vi "niFPGA Resampler Output Buffer.vi"(8 "wrEn":bool, 9 "wrVal":fxp<+/-,18,1>, 10 "ready for output":bool, 11 "reset":bool) -> (0 "wrTimedOut?":bool, 1 "rdTimedOut?":bool, 2 "outputValid":bool, 3 "outputData":fxp<+/-,18,1> format="%.18g")   [LabVIEW 2017]
uses:
  <vilib>/rvi/Emulation/niFpgaSctlEmulationGetInTimedLoop.vi
  <vilib>/Utility/error.llb/Clear Errors.vi
  <vilib>/rvi/DataTransferAndStorage/Container/Common/niFpgaContainerGetUniqueNameForEmu.vi
  <vilib>/rvi/DataTransferAndStorage/Container/Common/niFpgaContainerSetEmuInfo.vi
  <vilib>/rvi/eio/common/nirviEmuReportErrorAndStop.vi
  <vilib>/rvi/DataTransferAndStorage/Container/Common/niFpgaContainerExecOnDevCompGetState.vi
  <vilib>/rvi/Emulation/niFpgaEmulationIsFPGAContextNoSignature.vi
  <vilib>/rvi/errors/niFpgaSetErrorForExecOnDevCompSimple.vi
  <vilib>/rvi/FIFO/Fifo_Resource/nirvififoEmulationSetSize.vi
  <vilib>/rvi/FIFO/Fifo_Resource/nirviFifoEmulationQueueMgr.vi
  <instcachedir>/0/nirviFifoEmulationQueueMgr_E5CAEC123FF24DC58D834DCA3CDAA9B5.lvgen/nirviFifoEmulationQueueMgr_E5CAEC123FF24DC58D834DCA3CDAA9B5_002.vi
  <vilib>/rvi/FIFO/Fifo_Resource/nirvififoEmulationDetermineInputValidOut.vi
  <vilib>/rvi/FIFO/Fifo_Resource/nirvififoEmulationCreateLock.vi
  <vilib>/rvi/Emulation/niFpgaProcessEmulError.vi
  <vilib>/rvi/FIFO/Fifo_Resource/nirvififoEmulationObtainLock.vi
  <vilib>/rvi/FIFO/Fifo_Resource/nirvififoEmulationReleaseLock.vi
  <vilib>/rvi/occurrence/nirviWaitOnOccurrenceBase.vi
  <vilib>/rvi/errors/nirviReportUnexpectedCaseInternalError.vi
  <vilib>/rvi/errors/nirviReportUnexpectedCaseInternalError (U32).vi
  <vilib>/rvi/interface/RandomDataEmulation/niFpgaRandomDataHandleErrors.vi
  <vilib>/rvi/LocalResourceManager/LocalResourceManager.xnode
  <vilib>/rvi/DataTransferAndStorage/Container/XNode/niFpgaContainer.xnode
  <vilib>/rvi/FIFO/Fifo_Resource/niFpgaFifoEmulationRefIn.vi
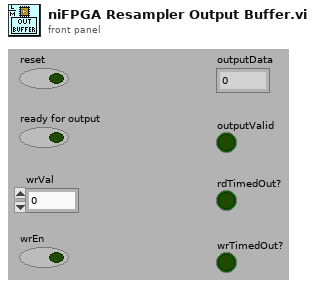
[diagram p1: front panel]
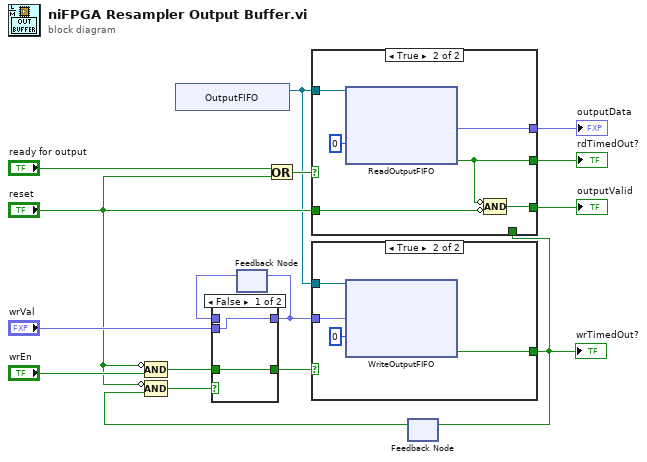
[diagram p0: block diagram]
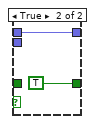
[diagram p2: hidden frame]
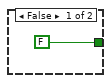
[diagram p3: hidden frame]
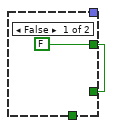
[diagram p4: hidden frame]
diagram:
  n1 = Compound Arithmetic op=AND(invert "reset", "wrEn") -> (w9:bool)
  n2 = xnode "OutputFIFO"() -> ("FIFO Out"=w3:refnum<k21>)
  n3 = feedback #1() -> (w14:fxp<+/-,18,1>)  [unwired: 1 out]
  n4 = Or(x="ready for output", y="reset") -> (x .or. y?=w6:bool)
  n5 = feedback #2() -> (w8:bool)  [unwired: 1 out]
  n6 = Compound Arithmetic op=AND(invert "reset", w8) -> (w7:bool)
  n7 = case shown="False" w7 {
    tunnel: [w17 w19] -> w12
    tunnel: "wrVal" -> [w17 _]
    tunnel: w9 -> [w18 _]
    tunnel: [w18 TRUE ("dataRDYOut")] -> w11
    tunnel: w14 -> [_ w19]
    frame False {
    }
    frame True {
    }
  }
  n8 = feedback-in #1(w12) -> ()
  n9 = case shown="True" w11 {
    tunnel: [FALSE ("Timed Out?") w24] -> w1
    tunnel: w12 -> [_ w23]
    tunnel: w3 -> [_ w22]
    frame False {
    }
    frame True {
      n10 = xnode "WriteOutputFIFO"("Element"=w23, "Timeout"=0, "FIFO In"=w22) -> ("Timed Out?"=w24:bool)  [unwired: 1 out]
    }
  }
  "wrTimedOut?" <- w1
  n11 = case shown="True" w6 {
    tunnel: [_ w31] -> w16
    tunnel: [w26 w30] -> w2
    tunnel: "reset" -> [_ w28]
    tunnel: [w26 w29] -> w15
    tunnel: w3 -> [_ w27]
    tunnel: w1 -> [_ _]
    frame False {
      w26 = FALSE
    }
    frame True {
      n12 = xnode "ReadOutputFIFO"("Timeout"=0, "FIFO In"=w27) -> ("Element"=w31:fxp<+/-,18,1>, "Timed Out?"=w29:bool)  [unwired: 1 out]
      n13 = Compound Arithmetic op=AND(invert w29, invert w28) -> (w30:bool)
    }
  }
  "outputData" <- w16
  "outputValid" <- w2
  "rdTimedOut?" <- w15
  n14 = feedback-in #2(w1) -> ()
